vi "MoveBySteps.vi"(0 "TranslationStage in":refnum<class "TranslationStagesInterface.lvclass">, 1 "Direction":enum16{"Forward", "Backwards"}(ring)=enum."Backwards", 5 "Steps":dbl, 7 "Channel":u16(ring)=1 items=["Channel1"=1, "Channel2"=2, "Channel3"=3, "Channel4"=4], 9 "Speed":u32, 11 "error in (no error)":errorcluster, 13 "Polarity":enum16{"Positive", "Negative"}(ring)) -> (4 "TranslationStage out":refnum<class "TranslationStagesInterface.lvclass">, 15 "error out":errorcluster)   [LabVIEW 2023, in "TranslationStage.lvlib" / "TranslationStagesInterface.lvclass"]
uses:
  TranslationStagesInterface.lvclass
panel:
  out "output cluster":T1
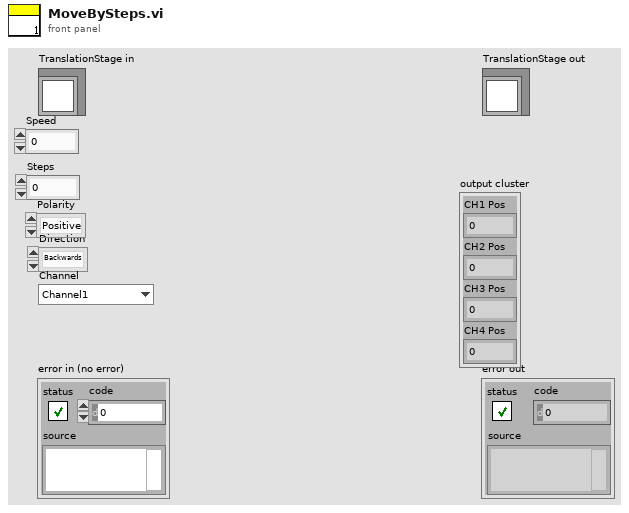
[diagram p1: front panel]
types:
  T1 = cluster{"CH1 Pos":i32, "CH2 Pos":i32, "CH3 Pos":i32, "CH4 Pos":i32}
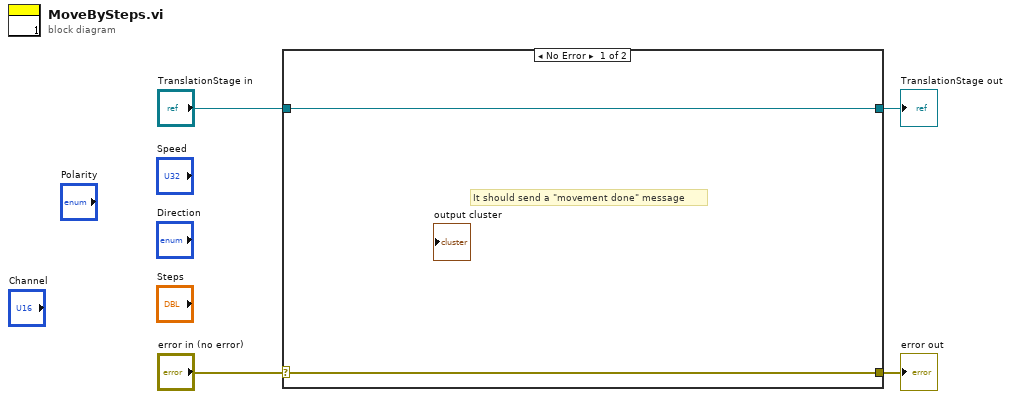
[diagram p0: block diagram]
diagram:
  n1 = case shown="No Error" "error in (no error)" {
    selector: "error in (no error)" -> [w5 w8]
    tunnel: [w5 w8] -> w3
    tunnel: [w6 w7] -> w1
    tunnel: "TranslationStage in" -> [w6 w7]
    frame No Error {
      # "It should send a \"movement done\" message"
    }
    frame Error {
    }
  }
  "error out" <- w3
  "TranslationStage out" <- w1
